vi "etlConversion01.vi"(1 "mode":u16(ring) items=["etl0 to 1", "etl1 to 0"], 2 "in":dbl) -> (0 "out":dbl)   [LabVIEW 2017]
uses:
  globalUtilities.vi
  <vilib>/Analysis/polynomials.llb/Scalar Polynomial Evaluation (DBL).vi
  <vilib>/Analysis/NI_AALPro.lvlib
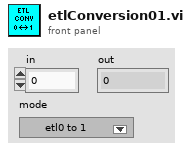
[diagram p1: front panel]
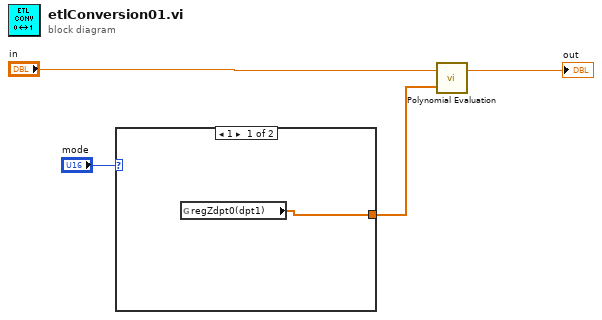
[diagram p0: block diagram]
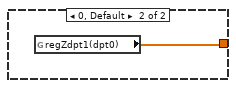
[diagram p2: hidden frame]
diagram:
  n1 = case shown="1" "mode" {
    tunnel: [w5 w6] -> w3
    frame 1 {
      n2 = global read "globalUtilities.vi" "regZdpt0(dpt1)"() -> (w5:dbl[])
    }
    frame 0, Default {
      n3 = global read "globalUtilities.vi" "regZdpt1(dpt0)"() -> (w6:dbl[])
    }
  }
  n4 = call-poly <vilib>:"Polynomial Evaluation.vi"("P(x)"=w3, "a"="in") -> ("P(a)"=→"out":dbl)  [unwired: 1 out]
